vi "Configure Start Trigger.vi"(0 "device session in":refnum<class "Device Session.lvclass">, 1 "trigger source":u8, 5 "trigger slope":T1, 7 "trigger level (V)":dbl, 9 "hysteresis level (V)":dbl, 11 "error in":errorcluster, 12 "start trigger type":enum8{"Software", "PFI0", "PXI Trig 0", "Edge"}(ring)) -> (4 "device session out":refnum<class "Device Session.lvclass">, 15 "error out":errorcluster)   [LabVIEW 2015, in "Device Session.lvclass"]
doc: "Configures the acquisition start trigger and in the case of an edge trigger, the selected channel source with the specified trigger level, hysteresis level and trigger slope. You must run the <B>Configure Channel</B> VI before running this VI.\n\n<B>Input Parameters</B>\n\n<B>device session in</B> is a reference to the session containing sessions to all instrument design libraries used in this sample project. This parameter is obtained from the 'Open Session' VI.\n\n<B>trigger source</B> specifies source to be monitored for edge trigger.\n\n<B>trigger slope</B> specifies either a positive slope or a negative slope for an edge trigger.\n\n<B>trigger level (V)</B> specifies the voltage threshold for the edge trigger.\n\n<B>hysteresis (V)</B> specifies the size of the hysteresis window on either side of the edge trigger level in volts. The digitizer triggers when the trigger signal passes through the hysteresis value you specify with this parameter, has the slope you specify with the trigger slope, and passes through the trigger level.\n\n<B>start trigger type</B> specifies which type of trigger to start an acquisition.\n\n<B>error in</B> describes error conditions that occur before this node runs. This input provides standard 'error in' functionality.\n\n<B>Output Parameters</B>\n\n<B>device session out</B> passes a reference to the session to the next VI.\n\n<B>error out</B> contains error information. This output provides standard 'error out' functionality."
uses:
  Device Session.lvclass
  <instrlib>/_niInstr/Data Trigger/v1/Shared/Public/Edge Configuration Trigger Slope.ctl
  Device Session.lvclass/Device Session.ctl
  FPGA Refnum.ctl
  <instrlib>/_niInstr/Data Trigger/v1/Shared/Public/Edge Configuration FXP(+-,18,1).ctl
  <vilib>/Utility/error.llb/Error Cluster From Error Code.vi
  <vilib>/rvi/errors/niLvFpgaAdjustHostInterfaceError.vi
  <vilib>/rvi/interface/nirviReadWriteControl/nirviReadWriteControl.xnode
  <instrlib>/_niInstr/Data Trigger/v1/Shared/niInstr Data Trigger v1 Shared.lvlib
  NiFpgaLv.dll
  <vilib>/rvi/interface/Simulation/niFpgaSimulationCallBeginRW.vi
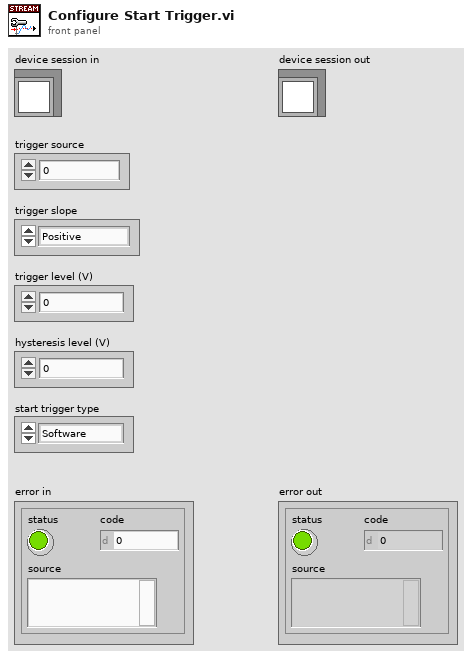
[diagram p1: front panel]
types:
  T1 = typedef "niInstr Data Trigger v1 Shared.lvlib/Edge Configuration Trigger Slope.ctl" = enum8{"Positive", "Negative"}
  T2 = typedef "niInstr Data Trigger v1 Shared.lvlib/Edge Configuration FXP(+-,18,1).ctl" = cluster{"highLevel":fxp<+/-,18,1>, "lowLevel":fxp<+/-,18,1>, "trigger slope":T1}
  T3 = typedef "Device Session.lvclass/FPGA Refnum.ctl" = refnum<k20>
  T4 = typedef "Device Session.lvclass/Device Session Object.ctl" = cluster{"ni5171R FPGA Reference":T3, "niHSAI config":refnum<class "niHSAI Config v1 Host.lvclass">, "configured scaling coefficients":cluster{"gain":dbl, "offset":dbl}[], "number of channels to stream":u8, "selected acq channels":bool[], "number of channels":u32, "actual channel configuration":T5[], "configured channels":bool[], "sample clock rate (Hz)":dbl}
  T5 = typedef "niHSAI Types v1 Host.lvlib/Channel Configuration.ctl" = cluster{"channel":u32, "coupling":T6, "impedance":T7, "bandwidth":T8, "vertical range":dbl, "vertical offset":dbl}
  T6 = typedef "niHSAI Types v1 Host.lvlib/Coupling.ctl" = enum8{"Default", "DC", "AC"}
  T7 = typedef "niHSAI Types v1 Host.lvlib/Impedance.ctl" = enum8{"Default", "1 mega ohm", "50 ohm"}
  T8 = typedef "niHSAI Types v1 Host.lvlib/Bandwidth.ctl" = enum8{"Default", "Full Bandwidth", "Anti-alias Filter"}
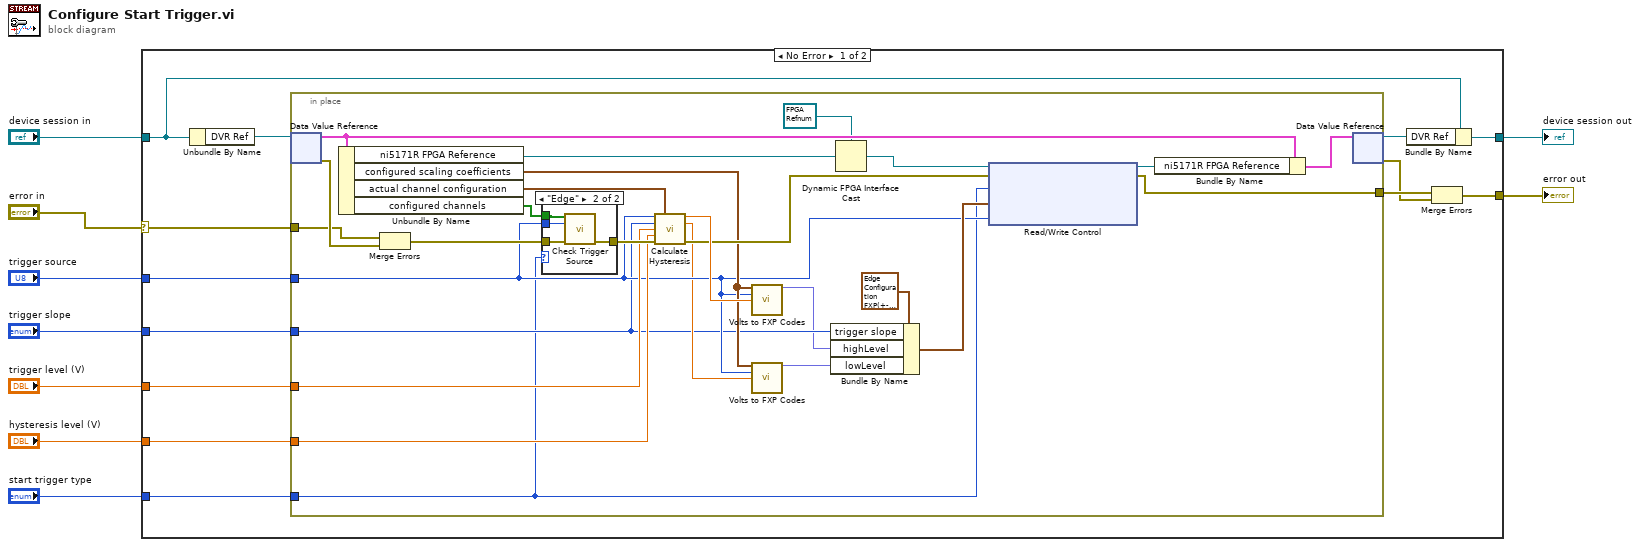
[diagram p0: block diagram]
diagram:
  n1 = case shown="No Error" "error in" {
    selector: "error in" -> [w22 w54]
    tunnel: "device session in" -> [w20 w55]
    tunnel: [w19 w55] -> w8
    tunnel: [w18 w54] -> w9
    tunnel: "start trigger type" -> [w17 _]
    tunnel: "trigger source" -> [w13 _]
    tunnel: "trigger level (V)" -> [w12 _]
    tunnel: "hysteresis level (V)" -> [w11 _]
    tunnel: "trigger slope" -> [w10 _]
    frame No Error {
      n2 = Unbundle By Name(w20) -> ("DVR Ref"=w21:refnum<data-value>)
      n3 = in-place {
        in-place-border: w22 -> [w46]
        in-place-border: [w44] -> w16
        in-place-border: w17 -> [w23]
        in-place-border: w13 -> [w28]
        in-place-border: w12 -> [w32]
        in-place-border: w11 -> [w33]
        in-place-border: w10 -> [w26]
        n4 = in-place-dvr #1(w21) -> (w48:T4, w47:errorcluster)
        n5 = Unbundle By Name(w48) -> ("ni5171R FPGA Reference"=w42:T3, "configured scaling coefficients"=w29:cluster{"gain":dbl, "offset":dbl}[], "actual channel configuration"=w34:T5[], "configured channels"=w37:bool[])
        n6 = Merge Errors(w46, w47) -> (w36:errorcluster)
        n7 = case shown="\"Edge\"" w23 {
          tunnel: w37 -> [_ w53]
          tunnel: w36 -> [w49 w52]
          tunnel: [w49 w51] -> w35
          tunnel: w28 -> [_ w50]
          frame Default {
          }
          frame "Edge" {
            n8 = call "Check Trigger Source.vi"("configured channels"=w53, "trigger source"=w50, "error in"=w52) -> ("error out"=w51:errorcluster)  [unwired: 12 in]
          }
        }
        n9 = call "Calculate Hysteresis.vi"("trigger source"=w28, "actual channel configuration"=w34, "trigger slope"=w26, "level (V)"=w32, "hysteresis (V)"=w33, "error in"=w35) -> ("high level (V)"=w31:dbl, "low level (V)"=w27:dbl, "error out"=w30:errorcluster)  [unwired: 7 in]
        n10 = call "Volts to FXP Codes.vi"("scaling coefficients"=w29, "channel index"=w28, "level (V)"=w31) -> ("codes"=w25:fxp<+/-,18,1>)  [unwired: 12 in]
        n11 = call "Volts to FXP Codes.vi"("scaling coefficients"=w29, "channel index"=w28, "level (V)"=w27) -> ("codes"=w24:fxp<+/-,18,1>)  [unwired: 12 in]
        n12 = Bundle By Name(cluster=T2 {"highLevel"=0.0, "lowLevel"=0.0, "trigger slope"=enum."Positive"} ("configuration"), "trigger slope"=w26, "highLevel"=w25, "lowLevel"=w24) -> (w38:T2)
        n13 = Dynamic FPGA Interface Cast(Session In=T3 refnum ("FPGA Interface"), Type=w42) -> (Session Out=w40:T3)
        n14 = xnode "Read/Write Control"("FPGA VI Reference In"=w40, "error in"=w30, "trig.start trigger select"=w23, "trig.trigger edge"=w38, "trig.edge trigger channel"=w28) -> ("FPGA VI Reference Out"=w45:T3, "error out"=w44:errorcluster)
        n15 = Bundle By Name(cluster=w48, "ni5171R FPGA Reference"=w45) -> (w43:T4)
        n16 = in-place-dvr #1(w43) -> (w14:refnum<data-value>, w15:errorcluster)
      }
      n17 = Bundle By Name(cluster=w20, "DVR Ref"=w14) -> (w19:refnum<class "Device Session.lvclass">)
      n18 = Merge Errors(w16, w15) -> (w18:errorcluster)
    }
    frame Error {
    }
  }
  "error out" <- w9
  "device session out" <- w8
